vi "InitAction.vi"(6 "InstrumentName":string, 7 "VisaRessIn":refnum<visa-resource-name>="GPIB0::12::INSTR", 8 "error in (no error)":errorcluster caption="entrée d'erreur (pas d'erreur)", 9 "FirstClassInst":bool, 10 "Function":string, 11 "EG_G5210 In":refnum<class "EG_G5210.lvclass"> caption="DNL_LabVIEW Object in") -> (0 "error out":errorcluster caption="sortie d'erreur", 3 "EG_G5210 Out":refnum<class "EG_G5210.lvclass"> caption="DNL_LabVIEW Object out")   [LabVIEW 2010, in "EG_G5210.lvclass"]
uses:
  EG_G5210.lvclass
  EG_G5210_Func.ctl
  EG_G5210.lvclass/EG_G5210.ctl
panel:
  in  "EG_G5210_Func":T1
  out "VisaRessOut":refnum<visa-resource-name>
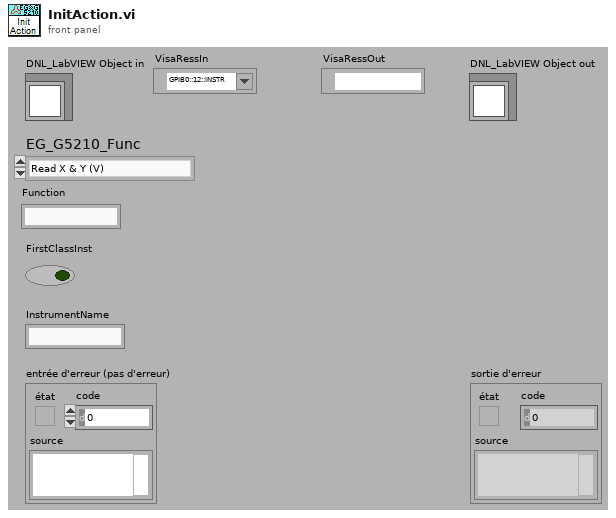
[diagram p1: front panel]
types:
  T1 = typedef "EG_G5210.lvclass/EG_G5210_Func.ctl" = enum16{"Read X & Y (V)", "Read Mag & Phase (V,°)", "Read X, Y, Mag & Phase (V,V,V,°)", "Read ADC Ch1 (V)", "Read ADC Ch2 (V)"}
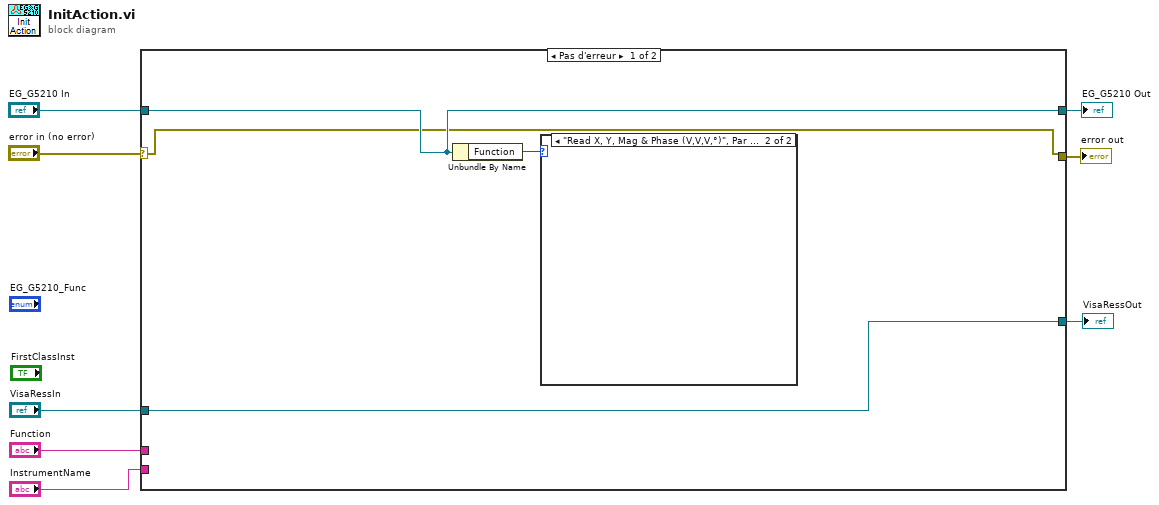
[diagram p0: block diagram]
diagram:
  n1 = case shown="Pas d'erreur" "error in (no error)" {
    selector: "error in (no error)" -> [w9 w14]
    tunnel: [w9 w14] -> w7
    tunnel: "EG_G5210 In" -> [w10 w13]
    tunnel: [w10 w13] -> w5
    tunnel: "Function" -> [_ _]
    tunnel: "VisaRessIn" -> [w11 _]
    tunnel: [w11 _] -> w2
    tunnel: "InstrumentName" -> [_ _]
    frame No Error {
      n2 = Unbundle By Name(w10) -> ("Function"=w12:T1)
      n3 = case shown="\"Read X, Y, Mag & Phase (V,V,V,°)\", Par défaut" w12 {
        frame "Read Mag & Phase (V,°)" {
        }
        frame "Read X, Y, Mag & Phase (V,V,V,°)", Default {
        }
      }
    }
    frame Error {
    }
  }
  "error out" <- w7
  "EG_G5210 Out" <- w5
  "VisaRessOut" <- w2
